vi "Mono.move.vi"(8 "Target position":dbl format="%#_13g", 9 "Current position":dbl format="%#_13g", 11 "VISA resource name":refnum<visa-resource-name>="Monochromator") -> (1 "done":bool)   [LabVIEW 2022 SP3]
panel:
  out "CMD":string
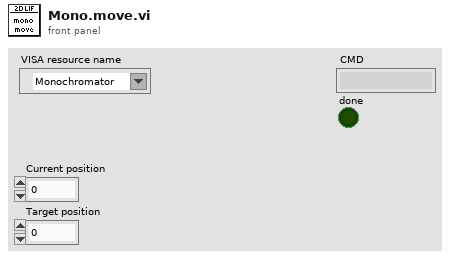
[diagram p1: front panel]
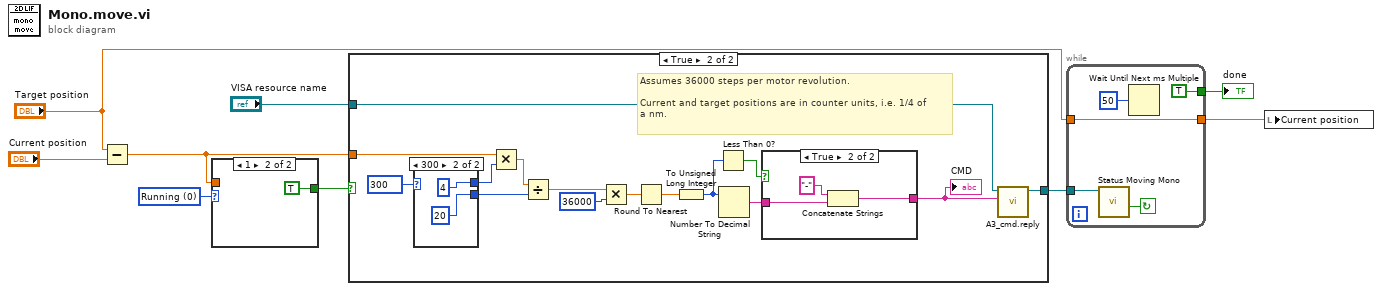
[diagram p0: block diagram]
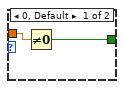
[diagram p2: hidden frame]
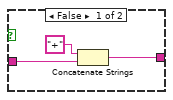
[diagram p4: hidden frame]
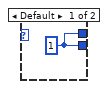
[diagram p5: hidden frame]
diagram:
  w1 = u16 0 items=["Running", "Testing"] ("Ring")
  n1 = Subtract(x="Target position", y="Current position") -> (x-y=w3:dbl)
  n2 = case shown="1" w1 {
    tunnel: [w11 TRUE] -> w8
    tunnel: w3 -> [w10 _]
    frame 0, Default {
      n3 = Not Equal To 0?(x=w10) -> (x != 0?=w11:bool)
    }
    frame 1 {
    }
  }
  n4 = case shown="True" w8 {
    tunnel: w3 -> [_ w24]
    tunnel: "VISA resource name" -> [w13 w26]
    tunnel: [w13 w25] -> w5
    frame False {
    }
    frame True {
      w19 = u16 300 items=["200"=200, "300"=300] ("Ring")
      # "Assumes 36000 steps per motor revolution.\n\nCurrent and target positions are in counter units, i.e. 1/4 of \na nm."
      n5 = case shown="300" w19 {
        tunnel: [w35 20] -> w22
        tunnel: [w35 4] -> w20
        frame Default {
          w35 = 1
        }
        frame 300 {
        }
      }
      n6 = Multiply(x=w24, y=w20) -> (x*y=w23:dbl)
      n7 = Divide(x=w23, y=w22) -> (x/y=w28:dbl)
      n8 = Multiply(x=w28, y=36000) -> (x*y=w16:dbl)
      n9 = Round To Nearest(number=w16) -> (nearest integer value=w15:dbl)
      n10 = To Unsigned Long Integer(number=w15) -> (unsigned 32bit integer=w14:u32)
      n11 = Less Than 0?(x=w14) -> (x < 0?=w27:bool)
      n12 = Number To Decimal String(number=w14) -> (decimal integer string=w18:string)  [unwired: 1 in]
      n13 = case shown="True" w27 {
        tunnel: [w30 w34] -> w17
        tunnel: w18 -> [w29 w32]
        frame False {
          n14 = Concatenate Strings("+", w29) -> (w30:string)
        }
        frame True {
          n15 = Concatenate Strings("-", w32) -> (w34:string)
        }
      }
      "CMD" <- w17
      n16 = call "A3_cmd.reply.vi"("cmd"=w17, "VISA resource name"=w26) -> ("VISA resource name out"=w25:refnum<visa-resource-name>)  [unwired: 7 in, 2 out]
    }
  }
  n17 = while {
    tunnel: w5 -> [w42]
    tunnel: [TRUE] -> w6
    tunnel: "Target position" -> [w38]
    tunnel: [w38] -> w4
    stop <- w40 continue-if-true
    n18 = call "Status Moving Mono.vi"("VISA resource name"=w42) -> ("moving?"=w40:bool)  [unwired: 9 in, 1 out]
    n19 = Wait Until Next ms Multiple(millisecond multiple=u32 50) -> ()  [unwired: 1 out]
  }
  "done" <- w6
  n20 = local write "Current position"(w4) -> ()
